vi "FGV.vi"(2 "Error In":errorcluster, 3 "Action":T5, 4 "Parameters In":T1={"Configuration"={"Table"=[], "Instrument"=[]}, "Startup Options"={"Door"=TRUE, "Curtain"=TRUE, "Pressure"=TRUE, "Turbo"=TRUE, "SysPoll"=TRUE, "GasFlag"=TRUE, "SourceExhaust"=TRUE}, "ADC Table"=[], "Q2 POL"=FALSE, "Q1 POL"=FALSE, "Simulation"=FALSE, "Exhsuast Gas Error"=FALSE, "Electronics ON"=FALSE, "Single Source"=FALSE, "L pump ON"=FALSE, "Laybold"=FALSE, "Ignore Error"=FALSE, "Scan Param"=FALSE, "Tuning Error"=FALSE, "RT Time"=0.0, "Error Msg"="", "Connected?"=FALSE, "Ready"=FALSE, "Fault"=FALSE}) -> (0 "Error Out":errorcluster, 1 "Parameters Out":T1={"Configuration"={"Table"=[], "Instrument"=[]}, "Startup Options"={"Door"=TRUE, "Curtain"=TRUE, "Pressure"=TRUE, "Turbo"=TRUE, "SysPoll"=TRUE, "GasFlag"=TRUE, "SourceExhaust"=TRUE}, "ADC Table"=[], "Q2 POL"=FALSE, "Q1 POL"=FALSE, "Simulation"=FALSE, "Exhsuast Gas Error"=FALSE, "Electronics ON"=FALSE, "Single Source"=FALSE, "L pump ON"=FALSE, "Laybold"=FALSE, "Ignore Error"=FALSE, "Scan Param"=FALSE, "Tuning Error"=FALSE, "RT Time"=0.0, "Error Msg"="", "Connected?"=FALSE, "Ready"=FALSE, "Fault"=FALSE})   [LabVIEW 2018]
uses:
  Type Defs/RT Parameters.ctl
  Type Defs/Main Configration.ctl
  Type Defs/Configration.ctl
  Type Defs/RT Configuration.ctl
  Type Defs/Global Action.ctl
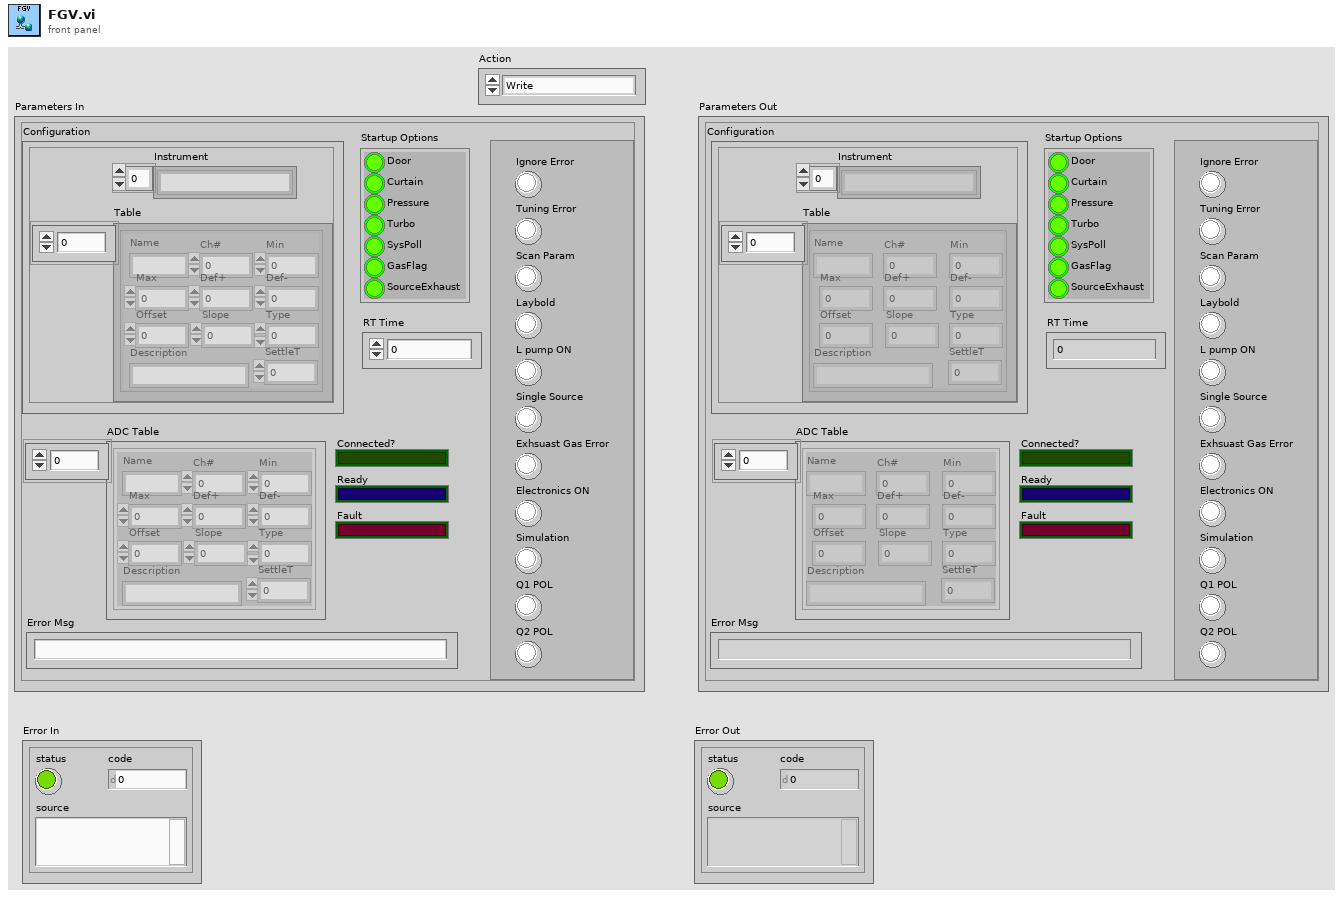
[diagram p1: front panel]
types:
  T1 = typedef "RT Parameters.ctl" = cluster{"Configuration":T2, "Startup Options":cluster{"Door":bool, "Curtain":bool, "Pressure":bool, "Turbo":bool, "SysPoll":bool, "GasFlag":bool, "SourceExhaust":bool}, "ADC Table":T4[], "Q2 POL":bool, "Q1 POL":bool, "Simulation":bool, "Exhsuast Gas Error":bool, "Electronics ON":bool, "Single Source":bool, "L pump ON":bool, "Laybold":bool, "Ignore Error":bool, "Scan Param":bool, "Tuning Error":bool, "RT Time":dbl, "Error Msg":string, "Connected?":bool, "Ready":bool, "Fault":bool}
  T2 = typedef "Main Configration.ctl" = cluster{"Table":T3[], "Instrument":string[]}
  T3 = typedef "Configration.ctl" = cluster{"Name":string, "Ch#":u8, "Min":dbl, "Max":dbl, "Def+":dbl, "Def-":dbl, "Offset":dbl, "Slope":dbl, "Type":u8, "Description":string, "SettleT":dbl}
  T4 = typedef "RT Configuration.ctl" = cluster{"Name":string, "Ch#":u8, "Min":dbl, "Max":dbl, "Def+":dbl, "Def-":dbl, "Offset":dbl, "Slope":dbl, "Type":u8, "Description":string, "SettleT":dbl}
  T5 = typedef "Global Action.ctl" = enum16{"Write", "Read"}
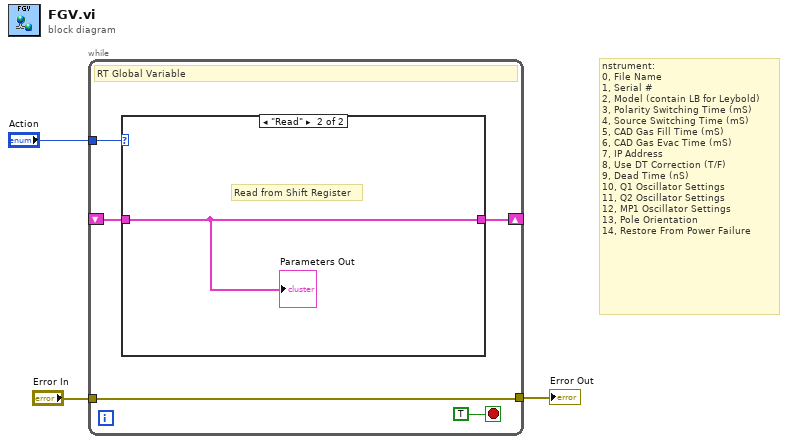
[diagram p0: block diagram]
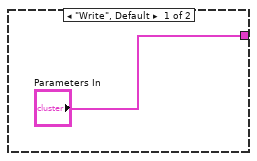
[diagram p2: hidden frame]
diagram:
  # "nstrument:\n0, File Name\n1, Serial #\n2, Model (contain LB for Leybold)\n3, Polarity Switching Time (mS)\n4, Source Switching Time (mS)\n5, CAD Gas Fill Time (mS)\n6, CAD Gas Evac Time (mS)\n7, IP Address\n8, Use DT Correction (T/F)\n9, Dead Time (nS)\n10, Q1 Oscillator Settings\n11, Q2 Oscillator Settings\n12, MP1 Oscillator Settings\n13, Pole Orientation\n14, Restore From Power Failure"
  n1 = while {
    tunnel: "Error In" -> [w7]
    tunnel: [w7] -> w2
    tunnel: "Action" -> [w6]
    shift-right: [w4] -> _
    shift-left: _ -> [w5]
    stop <- TRUE stop-if-true
    # "RT Global Variable"
    n2 = case shown="\"Read\"" w6 {
      tunnel: w5 -> [_ w10]
      tunnel: ["Parameters In" w10] -> w4
      frame "Write", Default {
      }
      frame "Read" {
        # "Read from Shift Register"
        "Parameters Out" <- w10
      }
    }
  }
  "Error Out" <- w2
